vi "Stop logic-Background MovCor.vi"(8 "error in":errorcluster) -> (0 "error out":errorcluster)   [LabVIEW 2017]
uses:
  Typedefs/Read Write Enum.ctl
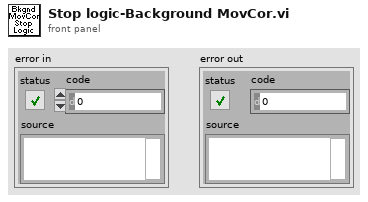
[diagram p1: front panel]
types:
  T1 = enum16{"Default", "Initialize", "Open", "Close", "Exit"}
  T2 = typedef "Read Write Enum.ctl" = enum16{"Read", "Write"}
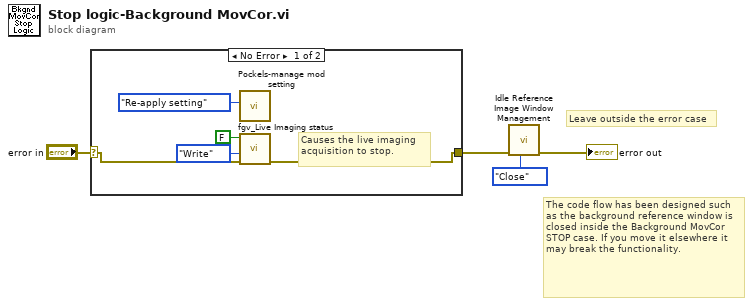
[diagram p0: block diagram]
diagram:
  # "The code flow has been designed such as the background reference window is closed inside the Background MovCor STOP case. If you move it elsewhere it may break the functionality."
  # "Leave outside the error case"
  n1 = case shown="No Error" "error in" {
    selector: "error in" -> [w5 w10]
    tunnel: [w6 w10] -> w1
    frame No Error {
      # "Causes the live imaging acquisition to stop."
      n2 = call "Pockels-manage mod setting.vi"("Function"=enum16{"Capture setting", "Re-apply setting"}."Re-apply setting") -> ()  [unwired: 10 in, 1 out]
      n3 = call "fgv_Live Imaging status.vi"("error in (no error)"=w5, "Function"=Read_Write_Enum."Write", "Live Imaging?"=FALSE ("Timelapse?")) -> ("error out"=w6:errorcluster)  [unwired: 7 in, 1 out]
    }
    frame Error {
    }
  }
  n4 = call "Idle Reference Image Window Management.vi"("Function"=T1."Close", "error in (no error)"=w1) -> ("error out"=→"error out":errorcluster)  [unwired: 9 in]
